vi "CRYMark Window Right.vi"() -> ()   [LabVIEW 2013]
uses:
  <vilib>/Utility/miscctls.llb/LVPositionTypeDef.ctl
  SubVI/CRYMain Sub Window Global.vi
panel:
  in  "sMe":string
  in  "bShow":bool=TRUE
  in  "Right":bool
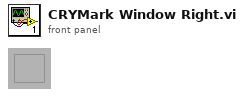
[diagram p1: front panel]
types:
  T1 = typedef "LVPositionTypeDef.ctl" = cluster{"Left":i32, "Top":i32}
  T2 = typedef "LVRectTypeDef.ctl" = cluster{"Left":i16, "Top":i16, "Right":i16, "Bottom":i16}
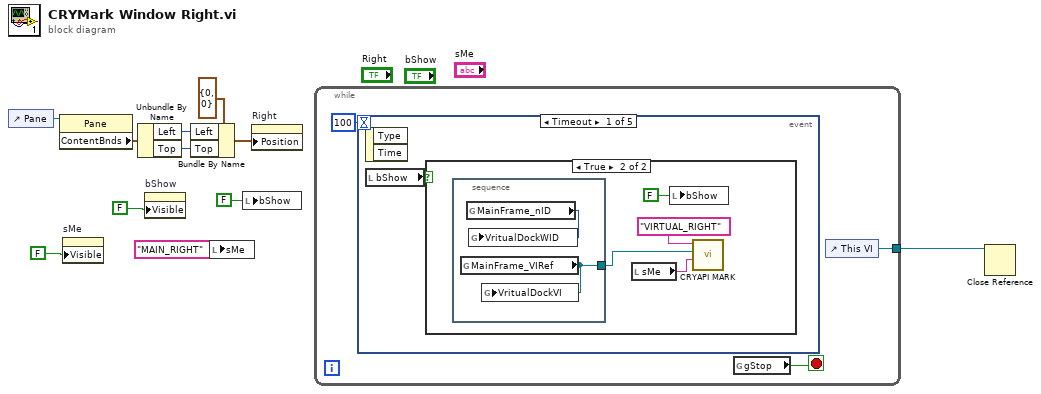
[diagram p0: block diagram]
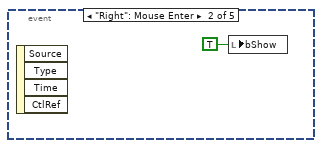
[diagram p3: hidden frame]
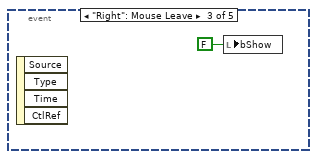
[diagram p4: hidden frame]
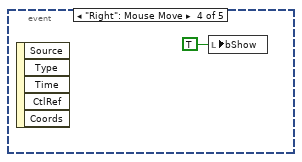
[diagram p5: hidden frame]
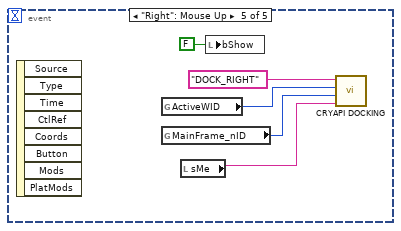
[diagram p6: hidden frame]
diagram:
  n1 = control-ref of="Pane"() -> (w11:refnum<vi>)
  n2 = property class="Pane"(reference=w11) -> ("ContentBnds"=w10:T2)  [unwired: 1 in, 2 out]
  n3 = property on="sMe" class="Str"("Visible"=FALSE) -> ()  [unwired: 2 in, 2 out]
  n4 = Unbundle By Name(w10) -> ("Left"=w9:i16, "Top"=w7:i16)
  n5 = property on="bShow" class="Bool (strict)"("Visible"=FALSE) -> ()  [unwired: 2 in, 2 out]
  n6 = Bundle By Name(cluster=T1 {"Left"=0, "Top"=0} ("Position"), "Left"=w9, "Top"=w7) -> (w6:T1)
  n7 = local write "sMe"("MAIN_RIGHT" ("sMe")) -> ()
  n8 = local write "bShow"(FALSE ("bShow")) -> ()
  n9 = property on="Right" class="Bool (strict)"("Position"=w6) -> ()  [unwired: 2 in, 2 out]
  n10 = while {
    tunnel: [w12] -> w1
    stop <- w13 stop-if-true
    n11 = event shown="[0] Timeout" {
      selector: _ -> [_ _ _ _ _]
      dyn-events: _ -> [_ _ _ _ _]
      timeout: 100 -> [_ _ _ _ _]
      event Timeout {
        n12 = event-data() -> ()  [unwired: 3 out]
        n13 = local read "bShow"() -> (w15:bool)
        n14 = case shown="True" w15 {
          frame False {
          }
          frame True {
            n15 = stacked-sequence {
              tunnel: [w20] -> w17
              frame #0 {
                n16 = global read "CRYMain Sub Window Global.vi" "MainFrame_VIRef"() -> (w20:refnum<vi>)
                n17 = global read "CRYMain Sub Window Global.vi" "MainFrame_nID"() -> (w21:i32)
                n18 = global write "CRYMain Sub Window Global.vi" "VritualDockWID"(w21) -> ()
                n19 = global write "CRYMain Sub Window Global.vi" "VritualDockVI"(w20) -> ()
              }
            }
            n20 = local read "sMe"() -> (w16:string)
            n21 = local write "bShow"(FALSE ("bShow")) -> ()
            n22 = call "CRYAPI MARK.vi"("sAction"="VIRTUAL_RIGHT" ("Action"), "mVritual_VIRef"=w17, "sData"=w16) -> ()  [unwired: 1 in, 7 out]
          }
        }
      }
      event "Right": Mouse Enter {
        n23 = event-data() -> ()  [unwired: 5 out]
        n24 = local write "bShow"(TRUE ("bShow")) -> ()
      }
      event "Right": Mouse Leave {
        n25 = event-data() -> ()  [unwired: 5 out]
        n26 = local write "bShow"(FALSE ("bShow")) -> ()
      }
      event "Right": Mouse Move {
        n27 = event-data() -> ()  [unwired: 6 out]
        n28 = local write "bShow"(TRUE ("bShow")) -> ()
      }
      event "Right": Mouse Up {
        n29 = event-data() -> ()  [unwired: 9 out]
        n30 = global read "CRYMain Sub Window Global.vi" "ActiveWID"() -> (w27:i32)
        n31 = global read "CRYMain Sub Window Global.vi" "MainFrame_nID"() -> (w26:i32)
        n32 = local read "sMe"() -> (w25:string)
        n33 = local write "bShow"(FALSE ("bShow")) -> ()
        n34 = call "CRYAPI DOCKING.vi"("sData"=w25, "nDWinID"=w26, "nSWinID"=w27, "sAction"="DOCK_RIGHT") -> ()  [unwired: 8 out]
      }
    }
    n35 = global read "CRYMain Sub Window Global.vi" "gStop"() -> (w13:bool)
    n36 = control-ref of="This VI"() -> (w12:refnum<vi>)
  }
  n37 = Close Reference(reference=w1) -> ()  [unwired: 1 in, 1 out]
